vi "processData.vi"(8 "error in (no error)":errorcluster, 10 "model":refnum<class "Model.lvclass">, 11 "EnabledState in":refnum<class "EnabledState.lvclass">) -> (0 "error out":errorcluster, 2 "model 2":refnum<class "Model.lvclass">, 3 "EnabledState out":refnum<class "EnabledState.lvclass">)   [LabVIEW 2013, in "EnabledState.lvclass"]
uses:
  EnabledState.lvclass
  Model/Model/Model.lvclass
  Typedefs/StateSelector.ctl
  Typedefs/M2AADTTypedefs.lvlib
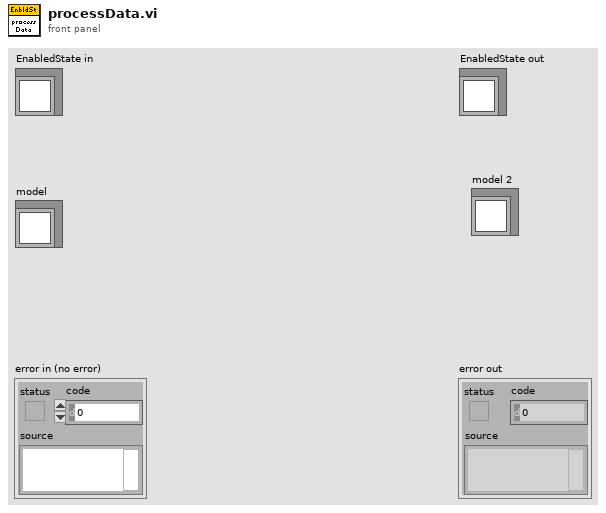
[diagram p1: front panel]
types:
  T1 = typedef "M2AADTTypedefs.lvlib/StateSelector.ctl" = enum16{"EndingCycleState", "FaultState", "InteractiveMotionState", "MovingToNewForceState", "OffState", "PausingState", "StandbyState", "StoppedState"}
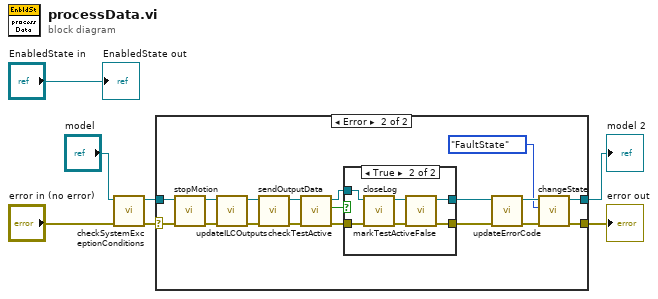
[diagram p0: block diagram]
diagram:
  n1 = call "checkSystemExceptionConditions.vi"("error in (no error)"="error in (no error)", "Model in"="model") -> ("error out"=w4:errorcluster, "Model out"=w3:refnum<class "Model.lvclass">)  [unwired: 8 in]
  n2 = case shown="Error" w4 {
    selector: w4 -> [w9 w21]
    tunnel: [w9 w25] -> w7
    tunnel: w3 -> [w8 w22]
    tunnel: [w8 w24] -> w5
    frame No Error {
    }
    frame Error {
      n3 = call "stopMotion.vi"("error in (no error)"=w21, "Model in"=w22) -> ("error out"=w11:errorcluster, "Model out"=w13:refnum<class "Model.lvclass">)  [unwired: 8 in]
      n4 = call "updateILCOutputs.vi"("error in (no error)"=w11, "Model in"=w13) -> ("error out"=w10:errorcluster, "Model out"=w12:refnum<class "Model.lvclass">)  [unwired: 8 in]
      n5 = call "sendOutputData.vi"("error in (no error)"=w10, "Model in"=w12) -> ("error out"=w14:errorcluster, "Model out"=w15:refnum<class "Model.lvclass">)  [unwired: 8 in]
      n6 = call "checkTestActive.vi"("error in (no error)"=w14, "Model in"=w15) -> ("error out"=w18:errorcluster, "testActiveIsTrue"=w20:bool, "Model out"=w19:refnum<class "Model.lvclass">)  [unwired: 7 in]
      n7 = case shown="True" w20 {
        tunnel: [w29 w32] -> w16
        tunnel: [w28 w30] -> w17
        tunnel: w19 -> [w29 w35]
        tunnel: w18 -> [w28 w34]
        frame False {
        }
        frame True {
          n8 = call "closeLog.vi"("error in (no error)"=w34, "Model in"=w35) -> ("error out"=w31:errorcluster, "Model out"=w33:refnum<class "Model.lvclass">)  [unwired: 8 in]
          n9 = call "markTestActiveFalse.vi"("error in (no error)"=w31, "Model in"=w33) -> ("error out"=w30:errorcluster, "Model out"=w32:refnum<class "Model.lvclass">)  [unwired: 8 in]
        }
      }
      n10 = call "updateErrorCode.vi"("error in (no error)"=w17, "Model in"=w16) -> ("error out"=w26:errorcluster, "Model out"=w27:refnum<class "Model.lvclass">)  [unwired: 8 in]
      n11 = call "changeState.vi"("error in (no error)"=w26, "State:"=StateSelector."FaultState", "Model in"=w27) -> ("error out"=w25:errorcluster, "Model out"=w24:refnum<class "Model.lvclass">)  [unwired: 7 in]
    }
  }
  "error out" <- w7
  "model 2" <- w5
  "EnabledState out" <- "EnabledState in"
